vi "Controlador_DAQ_PI.vi"() -> ()   [LabVIEW 2012]
panel:
  in  "Knob":dbl(knob) scale=0.0..5.0
  in  "Velocidad deseada\nRPM":dbl
  out "control ant":dbl
  out "error ant":dbl
  out "error":dbl
  out "Waveform Chart 2":dbl(graph)
  in  "stop":bool
  out "Waveform Chart":dbl(graph)
  in  "u_ini":dbl
  in  "error_ini":dbl
  # "MAX 3000"
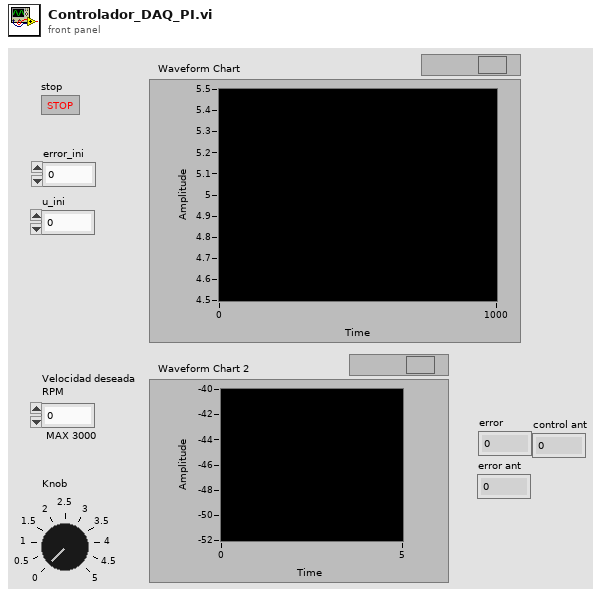
[diagram p1: front panel]
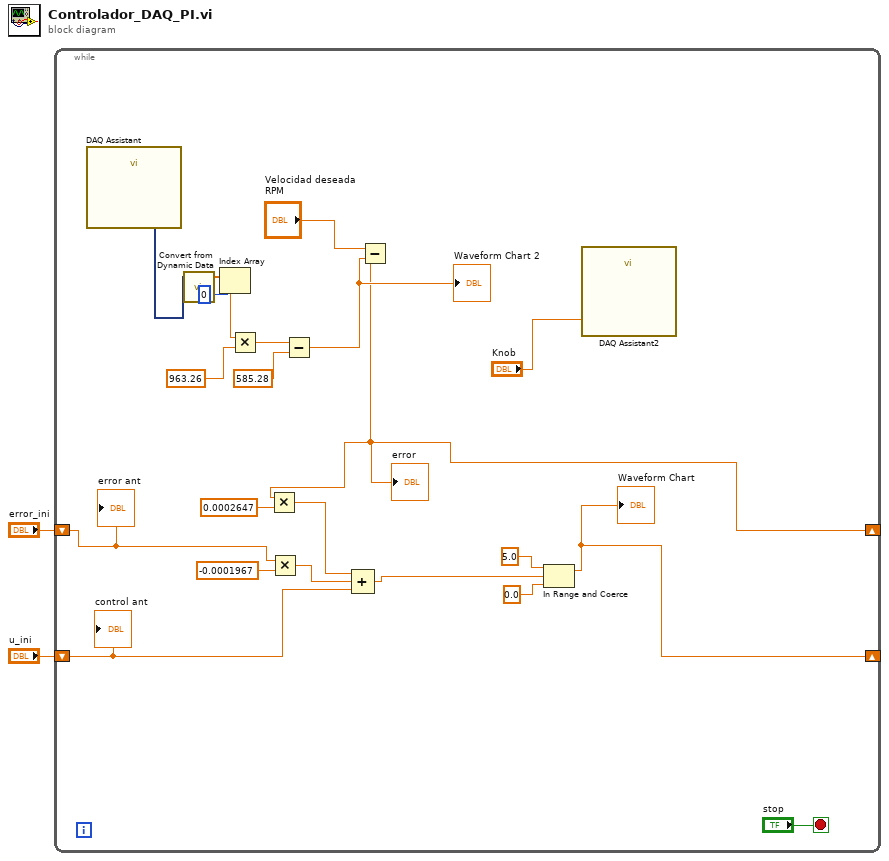
[diagram p0: block diagram]
diagram:
  n1 = while {
    shift-right: [w7] -> _
    shift-left: "error_ini" -> [w20]
    shift-right: [w4] -> _
    shift-left: "u_ini" -> [w19]
    stop <- "stop" stop-if-true
    n2 = call "DAQ Assistant"() -> ("data"=w5:dynamicdata)  [unwired: 17 in, 2 out]
    n3 = call "Convert from Dynamic Data"("Dynamic Data Type"=w5) -> ("Array"=w12:dbl[])  [unwired: 3 in]
    n4 = Index Array(array=w12, index=0) -> (element=w8:dbl)
    n5 = Multiply(x=w8, y=963.26) -> (x*y=w17:dbl)
    n6 = Multiply(x=w20, y=-0.0001967) -> (x*y=w24:dbl)
    n7 = Subtract(x=w17, y=585.28) -> (x-y=w9:dbl)
    "Waveform Chart 2" <- w9
    n8 = Subtract(x="Velocidad deseada\nRPM", y=w9) -> (x-y=w7:dbl)
    "error" <- w7
    n9 = Multiply(x=w7, y=0.0002647) -> (x*y=w23:dbl)
    n10 = Compound Arithmetic op=ADD(w23, w24, w19) -> (w15:dbl)
    n11 = In Range and Coerce(upper limit=5.0, x=w15, lower limit=0.0) -> (coerced(x)=w4:dbl)  [unwired: 1 out]
    "Waveform Chart" <- w4
    n12 = call "DAQ Assistant2"("data"="Knob") -> ()  [unwired: 17 in, 2 out]
    "error ant" <- w20
    "control ant" <- w19
  }
